vi "MPM_Get_Mode.vi"(8 "error in (no error)":errorcluster, 11 ".NET Reference in":refnum<k24>) -> (0 "error out":errorcluster, 2 "mode":i32(ring) items=["ManualRangeConstant", "ManualRangeSweep", "AutoRangeConstant", "AutoRangeSweep", "Freerun"], 3 "Reference out":refnum<k24>)   [LabVIEW 2017]
uses:
  LV_IL_Sample/DLL/InstrumentDLL.dll
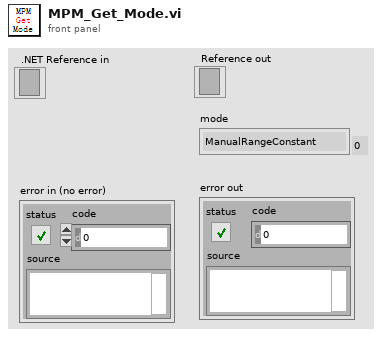
[diagram p1: front panel]
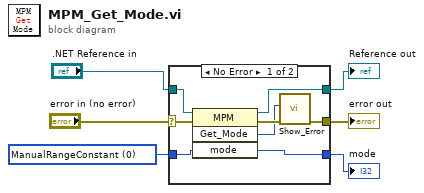
[diagram p0: block diagram]
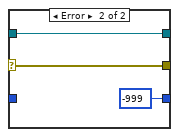
[diagram p2: hidden frame]
diagram:
  w4 = 0 items=["ManualRangeConstant", "ManualRangeSweep", "AutoRangeConstant", "AutoRangeSweep", "Freerun"] ("mode")
  n1 = case shown="No Error" "error in (no error)" {
    selector: "error in (no error)" -> [w10 w16]
    tunnel: [w14 -999 ("mode")] -> w1
    tunnel: ".NET Reference in" -> [w13 w17]
    tunnel: [w12 w17] -> w5
    tunnel: w4 -> [w11 _]
    tunnel: [w9 w16] -> w2
    frame No Error {
      n2 = invoke class="MPM" method="Get_Mode"(reference=w13, error in=w10, "mode"=w11) -> (reference out=w12:refnum<k24>, error out=w8:errorcluster, "Get_Mode"=w7:i32, "mode"=w14:i32)  [unwired: 1 in]
      n3 = call "Show_Error.vi"("error in (no error)"=w8, "Error"=w7) -> ("error out"=w9:errorcluster)  [unwired: 9 in]
    }
    frame Error {
    }
  }
  "Reference out" <- w5
  "error out" <- w2
  "mode" <- w1
